vi "OAT Torsional Vibration (Analog Tacho) (Waveform) (N Ch - N Settings).vi"(0 "analog tacho signals":waveform(dbl)[](array[waveform]), 1 "threshold (auto)":dbl[](array[numeric]), 2 "pulse/revolution (1)":i32[](array[numeric]) min=1, 3 "hysteresis (0)":dbl[](array[numeric]) format="%.2g", 4 "torsional vibration units":enum16{"RPM", "deg/s", "rad/s"}(ring), 5 "error in (no error)":errorcluster, 6 "missing pulses? (no:F)":bool[](array[boolean]), 7 "pulse width (2)":i32[](array[numeric]) min=0, 8 "reset? (F)":bool, 9 "slope (Rising)":u16[](array[ring]) items=["Rising", "Falling"], 10 "compensate geometric imperfection? (F)":bool, 11 "output interval [s]":dbl=0.001 min=0.0) -> (14 "torsional vibration signals":waveform(dbl)[](array[waveform]), 15 "speed profiles":T1[](array[typedef]) {"speed [RPM]" format="%.2f"; "time [s]" format="%.2f"}, 18 "unit labels":string[](array[string]), 19 "error out":errorcluster)   [LabVIEW 2017, in "SoundVib_Torsional.lvlib"]
doc: "Calculates torsional vibration signals from analog tachometer signals. This VI can return torsional vibration signals as either waveform signals or even-angle signals. Wire data to the <B>analog tacho signal</B> input to determine the polymorphic instance to use or manually select the instance."
uses:
  <vilib>/addons/Sound and Vibration/Order Analysis/Torsional Vibration/SoundVib_Torsional.lvlib
  <vilib>/addons/Sound and Vibration/Order Analysis/Tach Process/SubVIs/speed profile.ctl
  <vilib>/addons/_NISVFA/_Shared subVIs/Common/svc_Check for Waveform Parameter Continuity (no state).vi
  <vilib>/addons/_NISVFA/_Shared subVIs/Common/svc_Get SV Channel Info.vi
  <vilib>/addons/_NISVFA/_Shared subVIs/Common/svc_Engineering Units to Unit Label.vi
  <vilib>/addons/_NISVFA/_Shared subVIs/Common/svc_Unit Label to Engineering Units.vi
  <vilib>/addons/Sound and Vibration/Order Analysis/Tach Process/SoundVib_TachProcess.lvlib
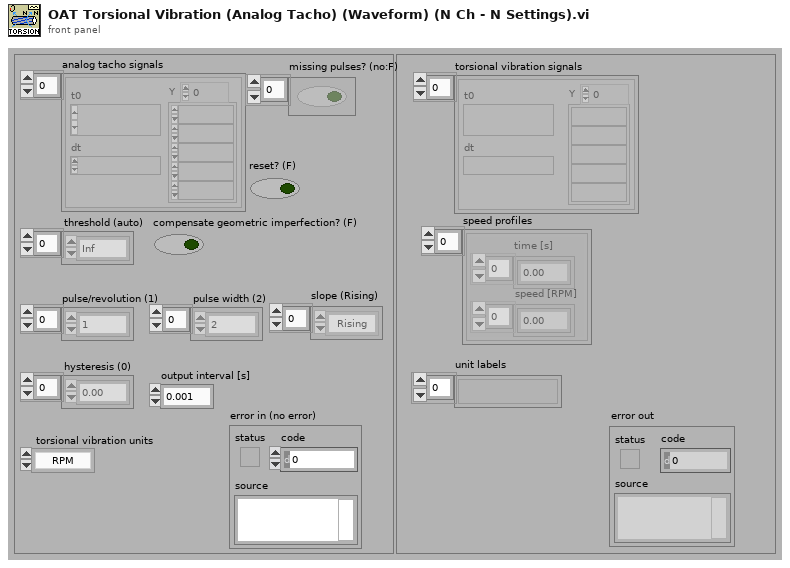
[diagram p1: front panel]
types:
  T1 = typedef "SoundVib_TachProcess.lvlib/speed profile.ctl" = cluster{"time [s]":dbl[], "speed [RPM]":dbl[]}
  T2 = cluster{"dt equal":bool, "array length equal":bool, "number channels change":bool}
  T3 = cluster{"dt":bool, "t0 continuity":bool, "array length":bool, "channel info":bool, "name":bool}
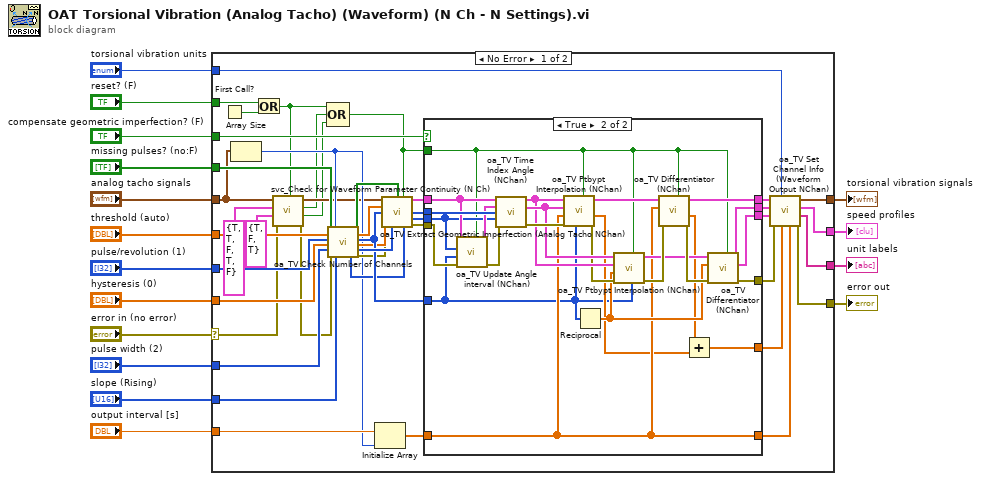
[diagram p0: block diagram]
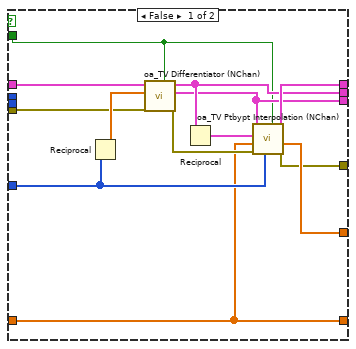
[diagram p2: hidden frame]
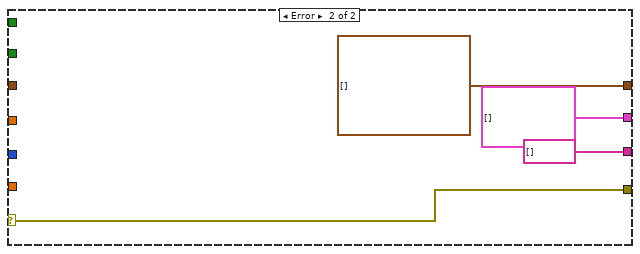
[diagram p3: hidden frame]
diagram:
  n1 = case shown="No Error" "error in (no error)" {
    selector: "error in (no error)" -> [w25 w102]
    tunnel: "threshold (auto)" -> [w54 _]
    tunnel: "pulse/revolution (1)" -> [w53 _]
    tunnel: "pulse width (2)" -> [w52 _]
    tunnel: "slope (Rising)" -> [w51 _]
    tunnel: "hysteresis (0)" -> [w32 _]
    tunnel: [w41 waveform(dbl)[] [] ("even time speed")] -> w7
    tunnel: [w42 w102] -> w12
    tunnel: "compensate geometric imperfection? (F)" -> [w35 _]
    tunnel: "reset? (F)" -> [w58 _]
    tunnel: "analog tacho signals" -> [w19 _]
    tunnel: "torsional vibration units" -> [w40 _]
    tunnel: [w38 T1[] [] ("speed profile")] -> w5
    tunnel: [w34 string[] [] ("unit labels")] -> w3
    tunnel: "missing pulses? (no:F)" -> [w30 _]
    tunnel: "output interval [s]" -> [w29 _]
    frame No Error {
      n2 = First Call?() -> (First Call?: T/F=w59:bool)
      n3 = Array Size(array=w19) -> (size(s)=w28:i32)
      n4 = Or(x=w58, y=w59) -> (x .or. y?=w23:bool)
      n5 = call <vilib>:"svc_Check for Waveform Parameter Continuity (N Ch).vi"("restart averaging (F)"=w23, "error in (no error)"=w25, "checks for multichannel parameters"=T2 {"dt equal"=TRUE, "array length equal"=FALSE, "number channels change"=TRUE}, "checks for channel parameter change"=T3 {"dt"=TRUE, "t0 continuity"=TRUE, "array length"=FALSE, "channel info"=TRUE, "name"=FALSE}, "scaled signal(s)"=w19) -> ("error out"=w24:errorcluster, "multichannel parameter changed"=w20:bool, "waveform parameter changed"=w21:bool, "dup scaled signal(s)"=w26:waveform(dbl)[])  [unwired: 3 out]
      n6 = Compound Arithmetic op=OR(w23, w21, w20) -> (w22:bool)
      n7 = call <vilib>:"oa_TV Check Number of Channels.vi"("missing pulses? (no:F)"=w30, "threshold (auto)"=w54, "pulse/revolution (1)"=w53, "hysteresis (0)"=w32, "pulse width (2)"=w52, "error in (no error)"=w24, "channel number"=w28, "slope (Rising)"=w51) -> ("slope out"=w46:u16[], "missing pulses? out"=w50:bool[], "threshold out"=w49:dbl[], "pulse/revolution out"=w47:i32[], "hysteresis out"=w33:dbl[], "pulse width out"=w48:i32[], "error out"=w31:errorcluster)  [unwired: 5 in]
      n8 = Initialize Array(w29, w28) -> (w27:dbl[])
      n9 = call <vilib>:"oa_TV Extract Geometric Imperfection (Analog Tacho NChan).vi"("analog tacho signal"=w26, "missing pulses? (no:F)"=w50, "reset? (F)"=w22, "threshold (auto)"=w49, "pulse/revolution"=w47, "hysteresis(0)"=w33, "error in (no error)"=w31, "pulse width (2)"=w48, "slope (Rising)"=w46) -> ("pulse positions"=w55:cluster{dbl[]}[], "revulotion"=w57:i32[], "revulotion index"=w56:i32[], "error out"=w60:errorcluster)  [unwired: 3 in]
      n10 = case shown="True" w35 {
        tunnel: w60 -> [w71 w80]
        tunnel: w57 -> [_ w81]
        tunnel: w56 -> [_ w75]
        tunnel: w55 -> [w73 w77]
        tunnel: w47 -> [w68 w76]
        tunnel: [w64 w91] -> w45
        tunnel: [w63 w90] -> w44
        tunnel: [w65 w89] -> w43
        tunnel: w27 -> [w66 w85]
        tunnel: [w67 w83] -> w39
        tunnel: [w62 w86] -> w37
        tunnel: [w66 w85] -> w36
        tunnel: w22 -> [w61 w74]
        frame False {
          n11 = Reciprocal(x=w68) -> (1/x=w72:dbl[])
          n12 = call <vilib>:"oa_TV Differentiator (NChan).vi"("reset? (False)"=w61, "error in (no error)"=w71, "delta X"=w72, "Y[n]"=w73) -> ("error out"=w69:errorcluster, "X[n]"=w62:cluster{dbl[]}[], "dY[n]/dX[n]"=w63:cluster{dbl[]}[])  [unwired: 4 in, 1 out]
          n13 = Reciprocal(x=w63) -> (1/x=w70:cluster{dbl[]}[])
          n14 = call <vilib>:"oa_TV Ptbypt Interpolation (NChan).vi"("reset? (F)"=w61, "buffer size"=w68, "error in (no error)"=w69, "dX"=w66, "Y"=w70, "X"=w62) -> ("error out"=w65:errorcluster, "X0"=w67:dbl[], "resampled Y"=w64:cluster{dbl[]}[])  [unwired: 2 in, 1 out]
        }
        frame True {
          n15 = call <vilib>:"oa_TV Update Angle interval (NChan).vi"("reset? (F)"=w74, "error in (no error)"=w80, "pulse/revolution"=w76, "revulotion index"=w75, "pulse position [s]"=w77) -> ("error out"=w79:errorcluster, "angle intervals"=w78:cluster{dbl[]}[])  [unwired: 5 in]
          n16 = call <vilib>:"oa_TV Time Index Angle (NChan).vi"("pulse positions"=w77, "angle intervals"=w78, "revulotion"=w81, "revulotion index"=w75, "error in (no error)"=w79) -> ("pulse positions"=w95:cluster{dbl[]}[], "angle"=w96:cluster{dbl[]}[], "error out"=w98:errorcluster)  [unwired: 8 in]
          n17 = call <vilib>:"oa_TV Ptbypt Interpolation (NChan).vi"("reset? (F)"=w74, "buffer size"=w76, "error in (no error)"=w98, "dX"=w85, "Y"=w96, "X"=w95) -> ("error out"=w94:errorcluster, "X0"=w84:dbl[], "resampled Y"=w97:cluster{dbl[]}[])  [unwired: 2 in, 1 out]
          n18 = Reciprocal(x=w76) -> (1/x=w88:dbl[])
          n19 = call <vilib>:"oa_TV Ptbypt Interpolation (NChan).vi"("reset? (F)"=w74, "buffer size"=w76, "error in (no error)"=w94, "dX"=w88, "Y"=w95, "X"=w96) -> ("error out"=w93:errorcluster, "resampled Y"=w87:cluster{dbl[]}[])  [unwired: 2 in, 2 out]
          n20 = call <vilib>:"oa_TV Differentiator (NChan).vi"("reset? (False)"=w74, "error in (no error)"=w93, "delta X"=w85, "Y[n]"=w97) -> ("error out"=w92:errorcluster, "Delay"=w82:dbl[], "dY[n]/dX[n]"=w91:cluster{dbl[]}[])  [unwired: 4 in, 1 out]
          n21 = Add(x=w82, y=w84) -> (x+y=w83:dbl[])
          n22 = call <vilib>:"oa_TV Differentiator (NChan).vi"("reset? (False)"=w74, "error in (no error)"=w92, "delta X"=w88, "Y[n]"=w87) -> ("error out"=w89:errorcluster, "X[n]"=w86:cluster{dbl[]}[], "dY[n]/dX[n]"=w90:cluster{dbl[]}[])  [unwired: 4 in, 1 out]
        }
      }
      n23 = call <vilib>:"oa_TV Set Channel Info (Waveform Output NChan).vi"("dt"=w36, "t0"=w39, "torisional vibration unit (RPM)"=w40, "error in (no error)"=w43, "pulse position"=w37, "seconds/revolution"=w44, "revolutions/minute"=w45) -> ("error out"=w42:errorcluster, "unit labels"=w34:string[], "speed profile"=w38:T1[], "torsional vibration"=w41:waveform(dbl)[])  [unwired: 1 in]
    }
    frame Error {
    }
  }
  "error out" <- w12
  "torsional vibration signals" <- w7
  "speed profiles" <- w5
  "unit labels" <- w3
